vi "Get Instrument Info.vi"(0 "RS NRPx Power Meter in":refnum<class "Power Meter.lvclass">, 11 "error in":errorcluster) -> (4 "RS NRPx Power Meter out":refnum<class "Power Meter.lvclass">, 15 "error out":errorcluster)   [LabVIEW 2023, in "RS NRPx Power Meter.lvlib" / "Power Meter.lvclass"]
uses:
  Power Meter.lvclass
  Instruments/Power Meter/Power Meter Base/Type Definitions/Instrument Info.ctl
  Instruments/Power Meter/Power Meter Base/Power Meter Base.lvclass/Power Meter Base.ctl
  Instruments/Power Meter/Power Meter Base/Properties/Write Instrument Info Array.vi
  <vilib>/nisyscfg/Find Hardware.vi
  <vilib>/nisyscfg/Close (System).vi
  <resource>/objmgr/niflexrioatomicsae.rc
  <vilib>/nisyscfg/nisyscfg.lvlib
  Instruments/Power Meter/Power Meter Base/Power Meter Base.lvclass
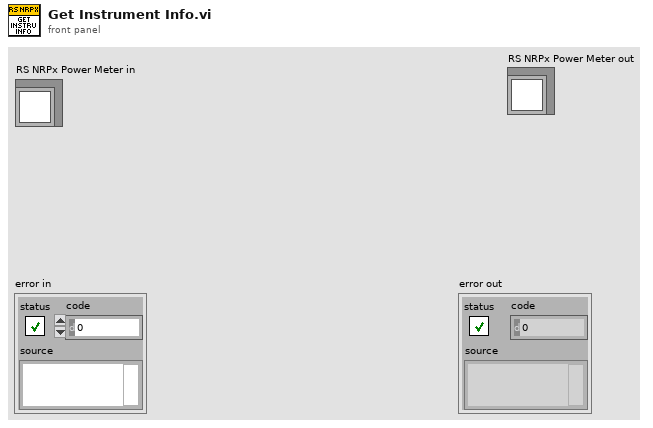
[diagram p1: front panel]
types:
  T1 = typedef "RFFixtureCharact.Instruments.lvlib/Power Meter Base.lvclass/Instrument Info.ctl" = cluster{"User Alias":string, "Resource Name":string, "Product Name":string, "Vendor Name":string}
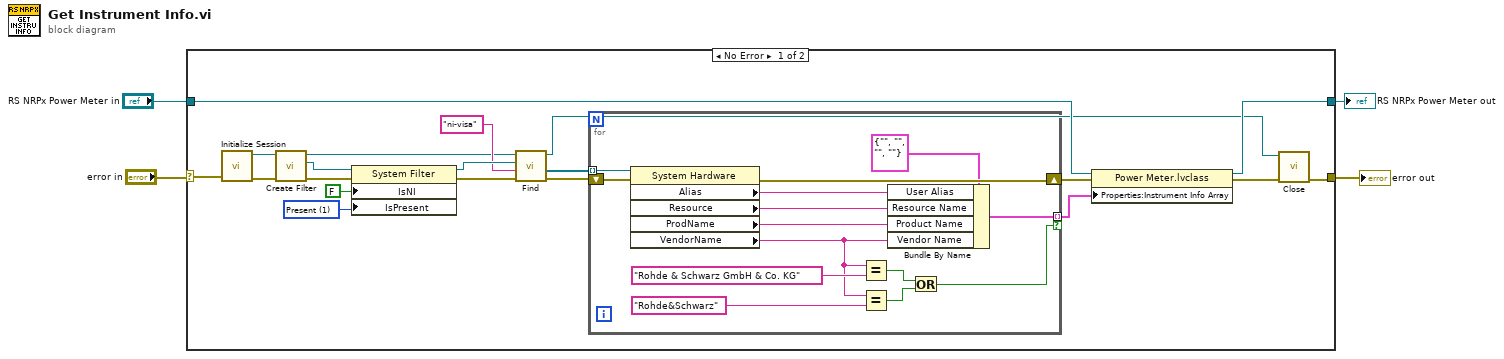
[diagram p0: block diagram]
diagram:
  n1 = case shown="No Error" "error in" {
    selector: "error in" -> [w15 w40]
    tunnel: [w11 w40] -> w4
    tunnel: "RS NRPx Power Meter in" -> [w8 w39]
    tunnel: [w7 w39] -> w1
    frame No Error {
      w14 = 1 items=["Unknown"=-1, "Not Present"=0, "Present"=1] ("Devices & Chassis:Is Present")
      n2 = call <vilib>:"Initialize Session.vi"("error in (no error)"=w15) -> ("error out"=w19:errorcluster, "Session out"=w21:refnum<k21>)  [unwired: 9 in]
      n3 = call <vilib>:"Create Filter.vi"("error in (no error)"=w19, "Session in"=w21) -> ("error out"=w24:errorcluster, "Filter out"=w16:refnum<k20>, "Session out"=w17:refnum<k21>)  [unwired: 7 in]
      n4 = property class="System Filter"(reference=w16, error in=w24, "IsNI"=FALSE ("Devices & Chassis:Is NI Product"), "IsPresent"=w14) -> (reference out=w23:refnum<k20>, error out=w22:errorcluster)
      n5 = call-poly <vilib>:"Find.vi"("error in (no error)"=w22, "Experts"="ni-visa", "Filter in"=w23, "Session in"=w17) -> ("error out"=w13:errorcluster, "Resources out"=w12:refnum<k20>[], "Session out"=w6:refnum<k21>)  [unwired: 4 in, 1 out]
      n6 = for {
        tunnel: w12 -> [w38] mode=indexing
        shift-right: [w37] -> w9
        shift-left: w13 -> [w36]
        tunnel: [w30] -> w5 mode=indexing if=w27
        n7 = property class="System Hardware"(reference=w38, error in=w36) -> (error out=w37:errorcluster, "Alias"=w33:string, "Resource"=w32:string, "ProdName"=w31:string, "VendorName"=w28:string)  [unwired: 1 out]
        n8 = Equal?(x=w28, y="Rohde & Schwarz GmbH & Co. KG") -> (x = y?=w26:bool)
        n9 = Equal?(x=w28, y="Rohde&Schwarz") -> (x = y?=w25:bool)
        n10 = Bundle By Name(cluster=T1 {"User Alias"="", "Resource Name"="", "Product Name"="", "Vendor Name"=""} ("Instrument Info Cluster"), "User Alias"=w33, "Resource Name"=w32, "Product Name"=w31, "Vendor Name"=w28) -> (w30:T1)
        n11 = Or(x=w26, y=w25) -> (x .or. y?=w27:bool)
      }
      n12 = property class="Power Meter.lvclass"(reference=w8, error in=w9, "Properties:Instrument Info Array"=w5) -> (reference out=w7:refnum<class "Power Meter.lvclass">, error out=w10:errorcluster)
      n13 = call-poly <vilib>:"Close.vi"("error in (no error)"=w10, "Session in"=w6) -> ("error out"=w11:errorcluster)  [unwired: 9 in]
    }
    frame Error {
    }
  }
  "error out" <- w4
  "RS NRPx Power Meter out" <- w1
